vi "ProcessName.vi"() -> (1 "ProcessName":string)   [LabVIEW 2017, in "Loop5.lvlib"]
uses:
  <vilib>/addons/InsightCM/Devices/Shared/Common/DataFlow/test/SpeedBenchmark/Loop5/Loop5.lvlib
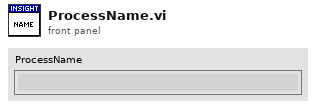
[diagram p1: front panel]
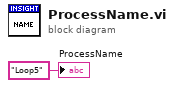
[diagram p0: block diagram]
diagram:
  "ProcessName" <- "Loop5" ("ProcessName")
